vi "Write LogSpec.vi"(8 "error in (no error)":errorcluster, 10 "data value":T1={"Log file folder"=path "C:/Users/NI/Desktop/Data", "Log file name"="LogFile_{Year}-{Month}-{Day}-{Hour}-{Minute}-{Second}.tdms", "Segment Files"=FALSE, "Segment File Size"=100} {"Segment File Size" format="%.0f MB"}, 11 "Performanced XNET CAN Signal Logger in":refnum<class "Performanced XNET CAN Logger.lvclass">) -> (0 "error out":errorcluster, 3 "Performanced XNET CAN Signal Logger out":refnum<class "Performanced XNET CAN Logger.lvclass">)   [LabVIEW 2021, in "Performanced XNET CAN Logger.lvlib" / "Performanced XNET CAN Logger.lvclass"]
uses:
  Performanced XNET CAN Logger.lvclass
  Typedef/Def-LogSpec.ctl
  Performanced XNET CAN Logger.lvclass/Performanced XNET CAN Logger.ctl
  XNET-CAN-Signal-Logger.lvlib
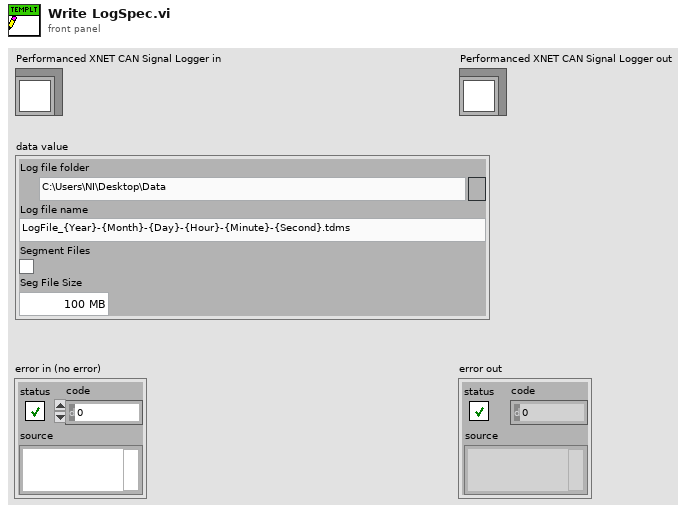
[diagram p1: front panel]
types:
  T1 = typedef "XNET-CAN-Signal-Logger.lvlib/Def-LogSpec.ctl" = cluster{"Log file folder":path, "Log file name":string, "Segment Files":bool, "Segment File Size":i64}
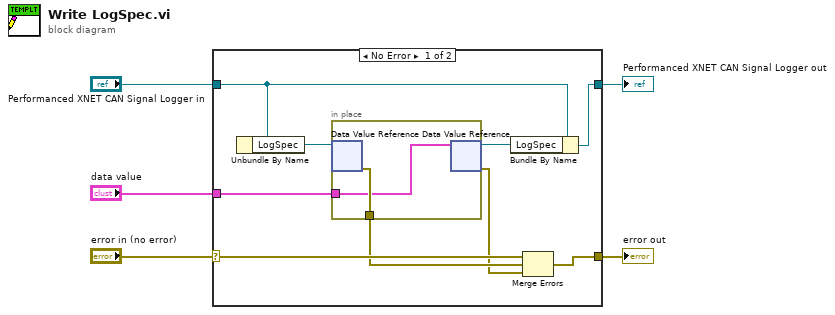
[diagram p0: block diagram]
diagram:
  n1 = case shown="No Error" "error in (no error)" {
    selector: "error in (no error)" -> [w14 w17]
    tunnel: [w9 w17] -> w4
    tunnel: [w13 w18] -> w2
    tunnel: "Performanced XNET CAN Signal Logger in" -> [w12 w18]
    tunnel: "data value" -> [w6 _]
    frame No Error {
      n2 = Unbundle By Name(w12) -> ("LogSpec"=w11:refnum<data-value>)
      n3 = in-place {
        in-place-border: [w16] -> w8
        in-place-border: w6 -> [w15]
        n4 = in-place-dvr #1(w11) -> (w16:errorcluster)  [unwired: 1 out]
        n5 = in-place-dvr #1(w15) -> (w10:refnum<data-value>, w7:errorcluster)
      }
      n6 = Bundle By Name(cluster=w12, "LogSpec"=w10) -> (w13:refnum<class "Performanced XNET CAN Logger.lvclass">)
      n7 = Merge Errors(w14, w8, w7) -> (w9:errorcluster)
    }
    frame Error {
    }
  }
  "error out" <- w4
  "Performanced XNET CAN Signal Logger out" <- w2
